vi "DestroyModuleBroadcasts.vi"(8 "error in (no error)":errorcluster, 11 "TesterModule in":refnum<class "TemplateModule.lvclass">) -> (0 "error out":errorcluster, 3 "TesterModule out":refnum<class "TemplateModule.lvclass">)   [LabVIEW 2024, in "TemplateModule.lvclass"]
uses:
  TemplateModule.lvclass
  TemplateModule.lvclass/TemplateModule.ctl
  JQMHCore/Module/RQMHModule.lvclass
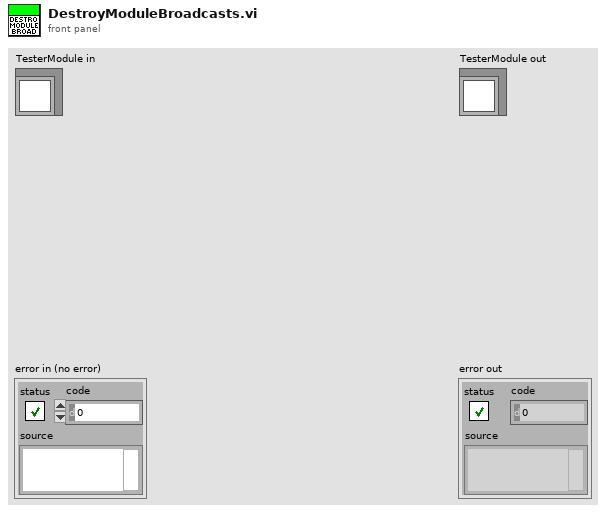
[diagram p1: front panel]
types:
  T1 = typedef "TemplateModule.lvclass/Broadcast Events--cluster.ctl" = cluster{"Stopped":refnum<user-event>, "NewControl258813080":refnum<user-event>, "NewControl260354259":refnum<user-event>}
  T2 = typedef "TemplateModule.lvclass/Request Events--cluster.ctl" = cluster{"Do Something":refnum<user-event>, "NewControl256895198":refnum<user-event>, "NewControl257342523":refnum<user-event>, "NewControl257429121":refnum<user-event>, "NewControl257700474":refnum<user-event>, "NewControl257813921":refnum<user-event>, "NewControl257861065":refnum<user-event>, "NewControl257971046":refnum<user-event>, "NewControl258050239":refnum<user-event>, "NewControl258223653":refnum<user-event>, "NewControl258270105":refnum<user-event>, "NewControl258297343":refnum<user-event>, "NewControl258480234":refnum<user-event>, "NewControl258517903":refnum<user-event>, "NewControl258631628":refnum<user-event>, "NewControl258654618":refnum<user-event>, "NewControl258691941":refnum<user-event>, "NewControl258844085":refnum<user-event>, "NewControl259026866":refnum<user-event>, "NewControl259125042":refnum<user-event>, "NewControl259500026":refnum<user-event>, "NewControl259578961":refnum<user-event>, "NewControl259604365":refnum<user-event>, "NewControl259661713":refnum<user-event>, "NewControl259709857":refnum<user-event>, "NewControl259844037":refnum<user-event>, "NewControl259980850":refnum<user-event>, "NewControl260104585":refnum<user-event>, "NewControl261112600":refnum<user-event>, "NewControl261693191":refnum<user-event>, "NewControl261831553":refnum<user-event>}
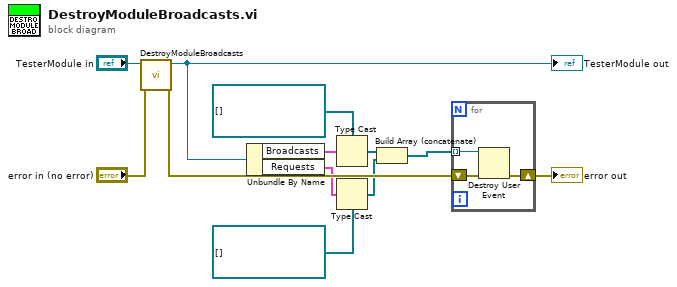
[diagram p0: block diagram]
diagram:
  n1 = call-parent "DestroyModuleBroadcasts.vi"("error in (no error)"="error in (no error)", "JQMHModule in"="TesterModule in") -> ("error out"=w6:errorcluster, "JQMHModule out"=w8:refnum<class "TemplateModule.lvclass">)  [unwired: 8 in]
  "TesterModule out" <- w8
  n2 = Unbundle By Name(w8) -> ("Broadcasts"=w11:T1, "Requests"=w4:T2)
  n3 = Type Cast(type=refnum<user-event>[] [] ("NewControl5"), x=w11) -> (*(type *) &x=w2:refnum<user-event>[])
  n4 = Type Cast(type=refnum<user-event>[] [] ("NewControl5"), x=w4) -> (*(type *) &x=w3:refnum<user-event>[])
  n5 = Build Array (concatenate)(w2, w3) -> (w1:refnum<user-event>[])
  n6 = for {
    tunnel: w1 -> [w15] mode=indexing
    shift-right: [w13] -> w10
    shift-left: w6 -> [w14]
    n7 = Destroy User Event(user event=w15, error in=w14) -> (error out=w13:errorcluster)
  }
  "error out" <- w10
